vi "Set square wave duty cycle (%).vi"(8 "error in (no error)":errorcluster, 10 "square wave duty cycle (%)":dbl=50.0 format="%0.2f", 11 "Generator in":refnum<class "Generador.lvclass">) -> (0 "error out":errorcluster, 3 "Generator out":refnum<class "Generador.lvclass">)   [LabVIEW 2020, in "FGen.lvlib" / "Generador.lvclass"]
uses:
  Generador.lvclass
  Generador.lvclass/Generador.ctl
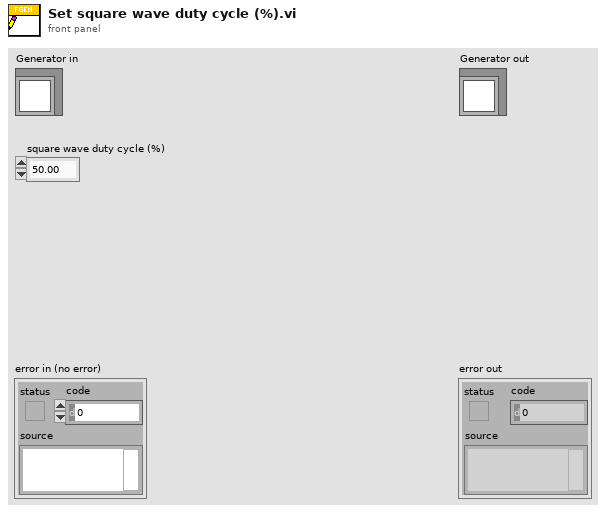
[diagram p1: front panel]
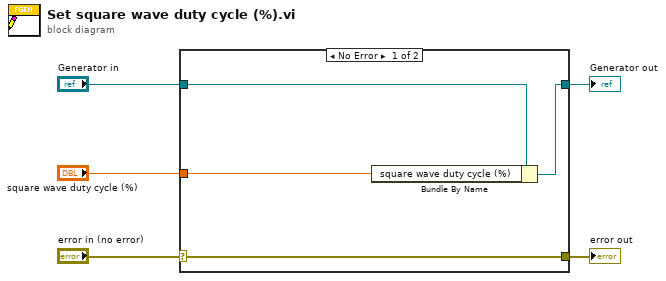
[diagram p0: block diagram]
diagram:
  n1 = case shown="No Error" "error in (no error)" {
    selector: "error in (no error)" -> [w9 w10]
    tunnel: [w9 w10] -> w4
    tunnel: [w7 w11] -> w2
    tunnel: "Generator in" -> [w8 w11]
    tunnel: "square wave duty cycle (%)" -> [w6 _]
    frame No Error {
      n2 = Bundle By Name(cluster=w8, "square wave duty cycle (%)"=w6) -> (w7:refnum<class "Generador.lvclass">)
    }
    frame Error {
    }
  }
  "error out" <- w4
  "Generator out" <- w2
